vi "Window Drag.vi"(8 "错误输入":errorcluster caption="错误输入（无错误）", 11 "last level":i32=1) -> (0 "错误输出":errorcluster)   [LabVIEW 2020]
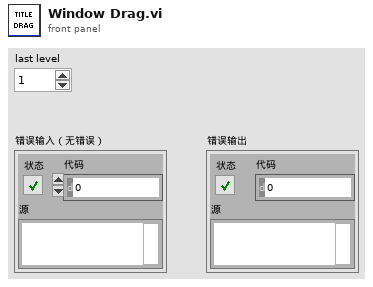
[diagram p1: front panel]
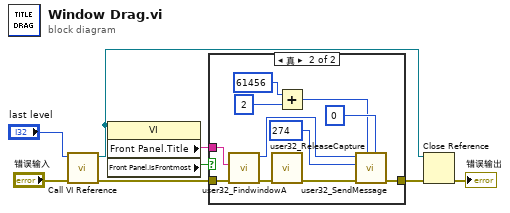
[diagram p0: block diagram]
diagram:
  n1 = call "Call VI Reference.vi"("error in"="错误输入", "last level"="last level") -> ("error out"=w3:errorcluster, "vi reference out"=w4:refnum<vi>)  [unwired: 8 in]
  n2 = property class="VI"(reference=w4) -> ("Front Panel.Title"=w8:string, "Front Panel.IsFrontmost"=w1:bool)  [unwired: 1 in, 2 out]
  n3 = case shown="真" w1 {
    tunnel: w8 -> [_ w20]
    tunnel: [w9 w11] -> w7
    tunnel: w3 -> [w9 w10]
    frame False {
    }
    frame True {
      n4 = call "user32_FindwindowA.vi"("error in (no error)"=w10, "lpWindowName"=w20) -> ("error out"=w13:errorcluster, "Return"=w12:u32)  [unwired: 8 in]
      n5 = call "user32_ReleaseCapture.vi"("error in (no error)"=w13) -> ("error out"=w14:errorcluster)  [unwired: 9 in, 1 out]
      n6 = Add(x=u32 61456, y=u32 2) -> (x+y=w18:u32)
      n7 = call "user32_SendMessage.vi"("IParam"=u32 0, "wParam"=w18, "error in (no error)"=w14, "Msg"=u32 274, "hWnd"=w12) -> ("error out"=w11:errorcluster)  [unwired: 5 in, 1 out]
    }
  }
  n8 = Close Reference(reference=w4, error in (no error)=w7) -> (error out=→"错误输出":errorcluster)
